vi "sub vi - Single Image.vi"(8 "Filename":string, 9 "yrange":dbl[](array[numeric]), 10 "xrange":dbl[](array[numeric]), 11 "save":bool) -> ()   [LabVIEW 2010]
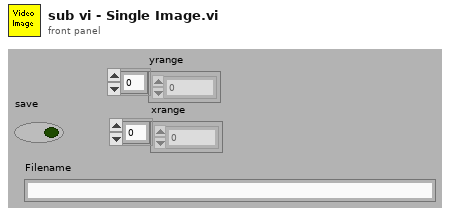
[diagram p1: front panel]
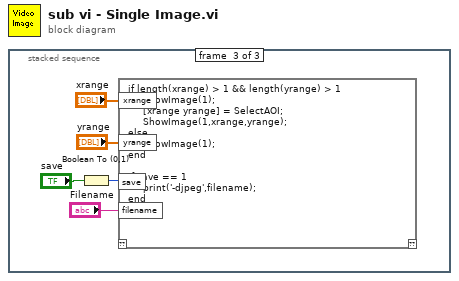
[diagram p0: block diagram]
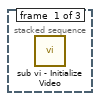
[diagram p2: hidden frame]
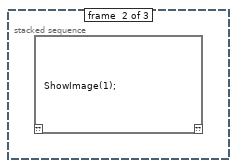
[diagram p3: hidden frame]
diagram:
  n1 = stacked-sequence {
    frame #0 {
      n2 = call "sub vi - Initialize Video.vi"() -> ()  [unwired: 1 out]
    }
    frame #1 {
      n3 = script code="ShowImage(1);"() -> ()  [unwired: 2 out]
    }
    frame #2 {
      n4 = Boolean To (0,1)(Boolean="save") -> (0, 1=w2:i16)
      n5 = script code="if length(xrange) > 1 && length(yrange) > 1\n     ShowImage(1);\n     [xrange yrange] = SelectAOI;\n     ShowImage(1,xrange,yrange);\nelse\n     ShowImage(1);\nend\n\nif save == 1\n     print('-djpeg',filename);\nend"("xrange"="xrange", "yrange"="yrange", "save"=w2, "filename"="Filename") -> ()  [unwired: 2 out]
    }
  }
